vi "Error Processor.vi"(8 "error in (no error)":errorcluster, 11 "Kasli Listener in":refnum<class "Kasli Listener.lvclass">) -> (0 "error out":errorcluster, 3 "Kasli Listener out":refnum<class "Kasli Listener.lvclass">)   [LabVIEW 2020, in "CIRCUS_uServices.lvlib" / "Kasli Listener and Writer.lvlib" / "Kasli Listener.lvclass"]
doc: "Use this VI to process all the error that are solvable inside this specific uService. Whatever is not possible to process, let it leave this VI and it will be processed by the Error Manager of the Distributed System."
uses:
  Kasli Listener.lvclass
  TALOS/TALOS_PPL.lvlibp/Internal uServices/System uServices/TCP Listener/TCP Listener/TCP Listener.lvclass
  TALOS/TALOS_PPL.lvlibp
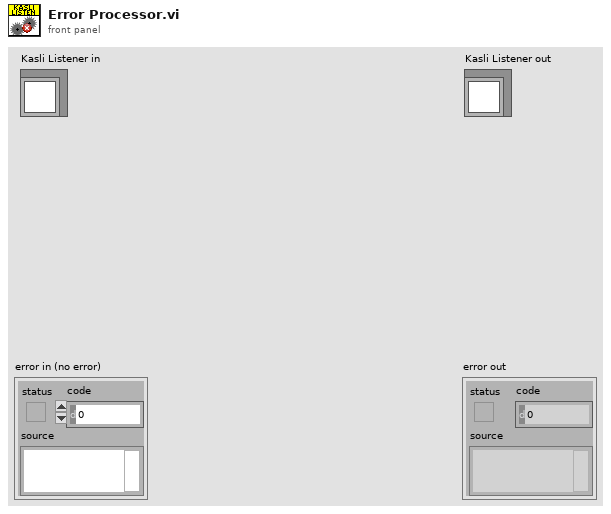
[diagram p1: front panel]
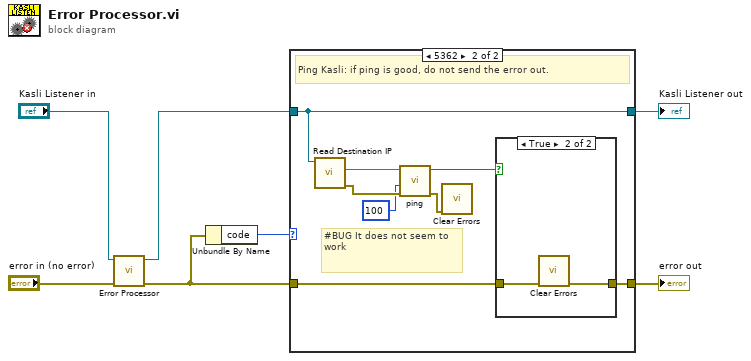
[diagram p0: block diagram]
diagram:
  n1 = call-parent "Error Processor.vi"("error in (no error)"="error in (no error)", "TCP Listener in"="Kasli Listener in") -> ("error out"=w1:errorcluster, "TCP Listener out"=w4:refnum<class "Kasli Listener.lvclass">)  [unwired: 8 in]
  n2 = Unbundle By Name(w1) -> ("code"=w2:i32)
  n3 = case shown="5362" w2 {
    tunnel: [w9 w15] -> w5
    tunnel: w4 -> [w9 w15]
    tunnel: w1 -> [w8 w17]
    tunnel: [w8 w16] -> w3
    frame Default {
      # "Let it through."
    }
    frame 5362 {
      # "#BUG It does not seem to work"
      # "Ping Kasli: if ping is good, do not send the error out."
      n4 = call-dynamic "Read Destination IP.vi"("TCP Listener in"=w15) -> ("error out"=w14:errorcluster, "Destination IP"=w12:string)  [unwired: 8 in, 1 out]
      n5 = call "ping.vi"("error in (no error)"=w14, "timeout (ms)"=100, "IP/Address"=w12) -> ("error out"=w10:errorcluster, "Success?"=w11:bool)  [unwired: 5 in, 2 out]
      n6 = call <vilib>:"Clear Errors.vi"("error in (no error)"=w10) -> ()  [unwired: 5 in, 2 out]
      n7 = case shown="True" w11 {
        tunnel: w17 -> [w18 w20]
        tunnel: [w18 w19] -> w16
        frame False {
        }
        frame True {
          n8 = call <vilib>:"Clear Errors.vi"("error in (no error)"=w20) -> ("error out"=w19:errorcluster)  [unwired: 5 in, 1 out]
        }
      }
    }
  }
  "error out" <- w3
  "Kasli Listener out" <- w5
